vi "Configure Parameter EDG.vi"(7 "PARAM":enum16{"TRAN", "SPE"}(ring), 8 "error in (no error)":errorcluster, 9 "speed（70 ps）":dbl=5e-11, 10 "STAT@TRAN":enum16{"RIS", "FALL"}(ring), 11 "VISA resource name":refnum<visa-resource-name>) -> (0 "error out":errorcluster, 3 "VISA resource name out":refnum<visa-resource-name>)   [LabVIEW 2018, in "Fluke 9500B.lvlib"]
uses:
  <instrlib>/Fluke 9500B/Fluke 9500B.lvlib
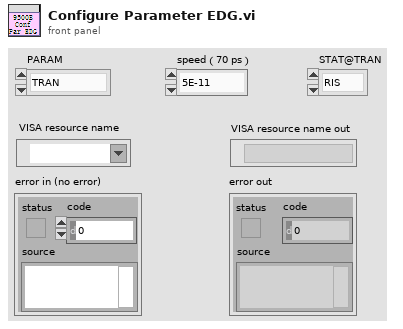
[diagram p1: front panel]
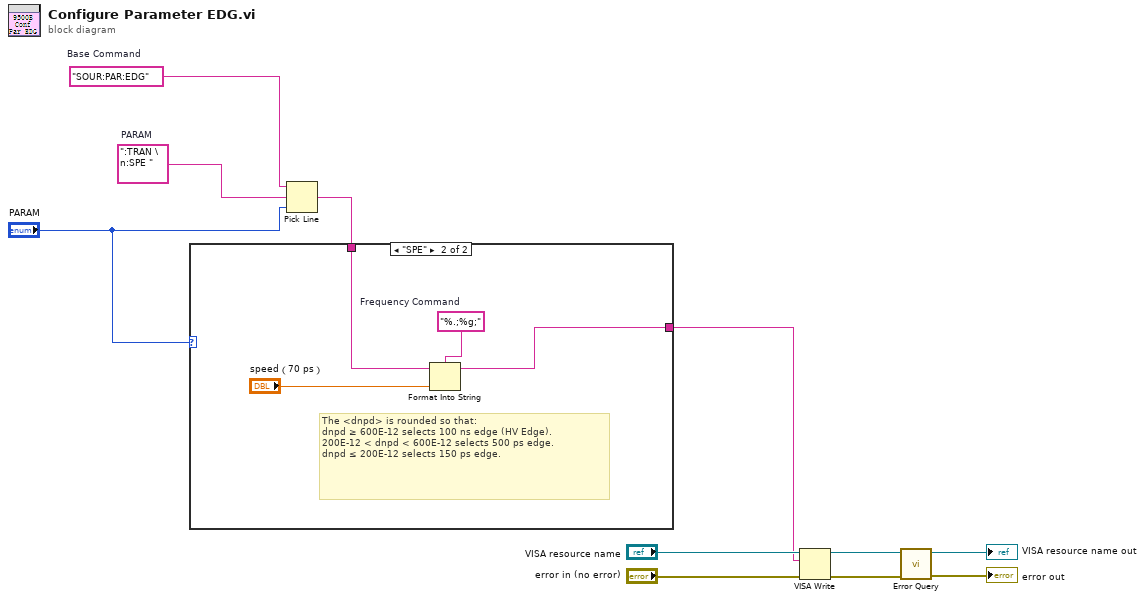
[diagram p0: block diagram]
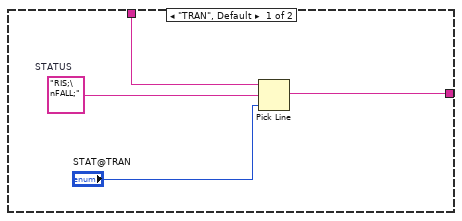
[diagram p2: hidden frame]
diagram:
  w8 = ":TRAN \n:SPE "  # PARAM
  w9 = "SOUR:PAR:EDG"  # Base Command
  n1 = Pick Line(string ("")=w9, multi-line string=w8, line index="PARAM") -> (output string=w7:string)
  n2 = case shown="\"SPE\"" "PARAM" {
    tunnel: w7 -> [w13 w18]
    tunnel: [w12 w16] -> w6
    frame "TRAN", Default {
      w15 = "RIS;\nFALL;"  # STATUS
      n3 = Pick Line(string ("")=w13, multi-line string=w15, line index="STAT@TRAN") -> (output string=w12:string)
    }
    frame "SPE" {
      w19 = "%.;%g;"  # Frequency Command
      # "The <dnpd> is rounded so that: \ndnpd ≥ 600E-12 selects 100 ns edge (HV Edge). \n200E-12 < dnpd < 600E-12 selects 500 ps edge. \ndnpd ≤ 200E-12 selects 150 ps edge."
      n4 = Format Into String(format string=w19, initial string=w18, "speed（70 ps）") -> (resulting string=w16:string)  [unwired: 1 in, 1 out]
    }
  }
  n5 = VISA Write(VISA resource name="VISA resource name", write buffer=w6, error in (no error)="error in (no error)") -> (VISA resource name out=w4:refnum<visa-resource-name>, error out=w3:errorcluster)  [unwired: 1 out]
  n6 = call <instrlib>:"Error Query.vi"("error in (no error)"=w3, "VISA resource name"=w4) -> ("error out"=→"error out":errorcluster, "VISA resource name out"=→"VISA resource name out":refnum<visa-resource-name>)  [unwired: 6 in, 2 out]
